vi "SPADQ_DeleteControlUnit.vi"(8 "error in":errorcluster, 10 "adq_cu_ptr":refnum<k24>, 11 "ADQAPI Ref":refnum<k24>) -> (0 "error out":errorcluster)   [LabVIEW 2022 SP3]
uses:
  C:/Windows/System32/ADQAPI_dotNet_helper.dll
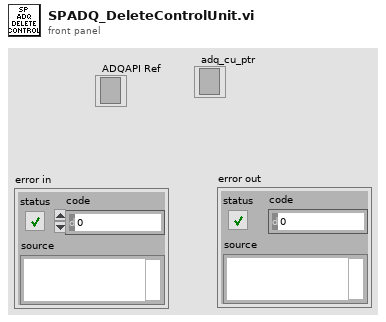
[diagram p1: front panel]
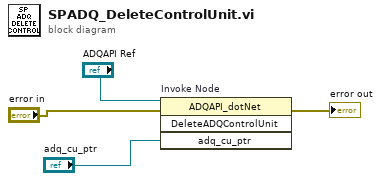
[diagram p0: block diagram]
diagram:
  n1 = invoke on="Invoke Node" class="ADQAPI_dotNet" method="DeleteADQControlUnit"(reference="ADQAPI Ref", error in="error in", "adq_cu_ptr"="adq_cu_ptr") -> (error out=→"error out":errorcluster)  [unwired: 1 in, 3 out]
